vi "Simple Sawtooth Waveform.vi"(6 "delta t":dbl=1.0, 7 "amplitude":dbl=1.0, 9 "n cycles":dbl=1.0, 10 "t0":dbl, 11 "offset":dbl) -> (3 "sawtooth waveform":waveform(dbl))   [LabVIEW 2023]
doc: "Produces a sawtooth wave."
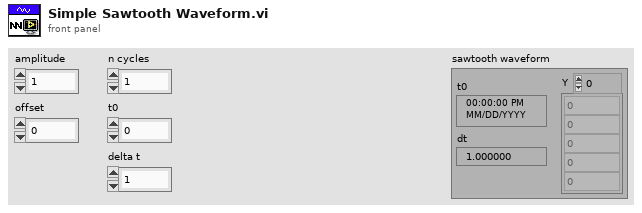
[diagram p1: front panel]
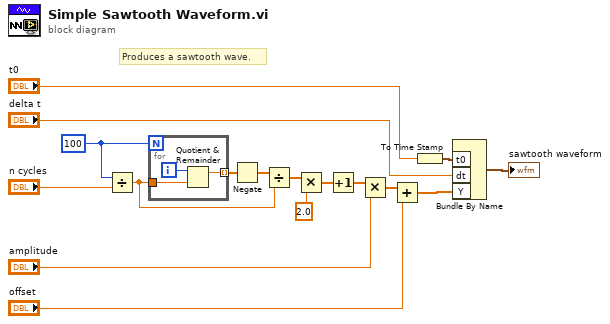
[diagram p0: block diagram]
diagram:
  w10 = 100 ("n points")
  # "Produces a sawtooth wave."
  n1 = Divide(x=w10, y="n cycles") -> (x/y=w4:dbl)
  n2 = for {
    N: w10 -> [_]
    tunnel: [w18] -> w8 mode=indexing
    tunnel: w4 -> [w19]
    i -> [w20]
    n3 = Quotient & Remainder(x=w20, y=w19) -> (x-y*floor(x/y)=w18:dbl)  [unwired: 1 out]
  }
  n4 = Negate(x=w8) -> (-x=w6:dbl[])
  n5 = Divide(x=w6, y=w4) -> (x/y=w5:dbl[])
  n6 = Multiply(x=w5, y=2.0) -> (x*y=w2:dbl[])
  n7 = Increment(x=w2) -> (x+1=w7:dbl[])
  n8 = Multiply(x=w7, y="amplitude") -> (x*y=w14:dbl[])
  n9 = Add(x=w14, y="offset") -> (x+y=w12:dbl[])
  n10 = To Time Stamp(1:"t0") -> (0:w3:timestamp)
  n11 = Bundle By Name("t0"=w3, "dt"="delta t", "Y"=w12) -> (→"sawtooth waveform":waveform(dbl))  [unwired: 1 in]
